vi "Load Reference.vi"(8 "error in (no error)":errorcluster, 10 "Reference":refnum<vi>, 11 "SingleStepTestV3 in":refnum<class "SingleStepTestV3.lvclass">) -> (0 "error out":errorcluster, 3 "SingleStepTestV3 out":refnum<class "SingleStepTestV3.lvclass">)   [LabVIEW 2022 SP3, in "SingleStepTestV3.lvlib" / "SingleStepTestV3.lvclass"]
doc: "The <b>Load Reference VI</b> is a dynamic dispatch VI that must be overwritten in every QControl Class and must <b>Call Parent Method</b>. This recursively loads the reference of the control to the data space for the Control Class up the inheritance hierarchy (class hierarchy). These references must be loaded in this way to use all of the built-in properties.\n\nThe reference input is the reference type needed for the control but is coerced to Generic. It should be cast back to the correct type before bundling into the class private data. The pre-casted \"Generic\" reference is wired as input to the <b>Call Parent Method</b>.\n<b> </b> <b> </b>\n©2016 Q Software Innovations, LLC (QSI)\nwritten by Quentin Alldredge\nproduced in LabVIEW 2015\n\nsupport@qsoftwareinnovations.com\nwww.qsoftwareinnovations.com\n\nAll rights reserved.\n\nRedistribution and use in source and binary forms, with or without modification, are permitted provided that the following conditions are met:\n\n * Redistributions of source code must retain the above copyright notice, this list of conditions and the following disclaimer.\n * Redistributions in binary form must reproduce the above copyright notice, this list of conditions and the following disclaimer in the documentation and/or other materials provided with the distribution.\n * Neither the name of Q Software Innovations, LLC. nor the names of its contributors may be used to endorse or promote products derived from this software without specific prior written permission.\n\nTHIS SOFTWARE IS PROVIDED BY THE COPYRIGHT HOLDERS AND CONTRIBUTORS \"AS IS\" AND ANY EXPRESS OR IMPLIED WARRANTIES, INCLUDING, BUT NOT LIMITED TO, THE IMPLIED WARRANTIES OF MERCHANTABILITY AND FITNESS FOR A PARTICULAR PURPOSE ARE DISCLAIMED. IN NO EVENT SHALL THE COPYRIGHT OWNER OR CONTRIBUTORS BE LIABLE FOR ANY DIRECT, INDIRECT, INCIDENTAL, SPECIAL, EXEMPLARY, OR CONSEQUENTIAL DAMAGES (INCLUDING, BUT NOT LIMITED TO, PROCUREMENT OF SUBSTITUTE GOODS OR SERVICES; LOSS OF USE, DATA, OR PROFITS; OR BUSINESS INTERRUPTION) HOWEVER CAUSED AND ON ANY THEORY OF LIABILITY, WHETHER IN CONTRACT, STRICT LIABILITY, OR TORT (INCLUDING NEGLIGENCE OR OTHERWISE) ARISING IN ANY WAY OUT OF THE USE OF THIS SOFTWARE, EVEN IF ADVISED OF THE POSSIBILITY OF SUCH DAMAGE."
uses:
  SingleStepTestV3.lvclass
  SingleStepTestV3.lvclass/SingleStepTestV3.ctl
  <vilib>/QSI/QControls/QControl Classes/Cluster/Cluster.lvclass
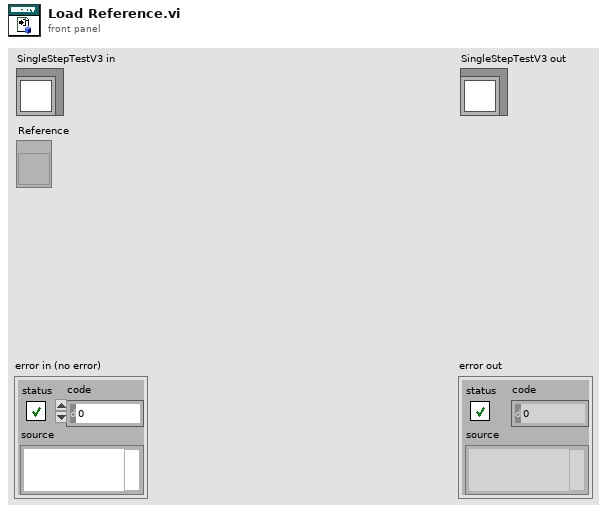
[diagram p1: front panel]
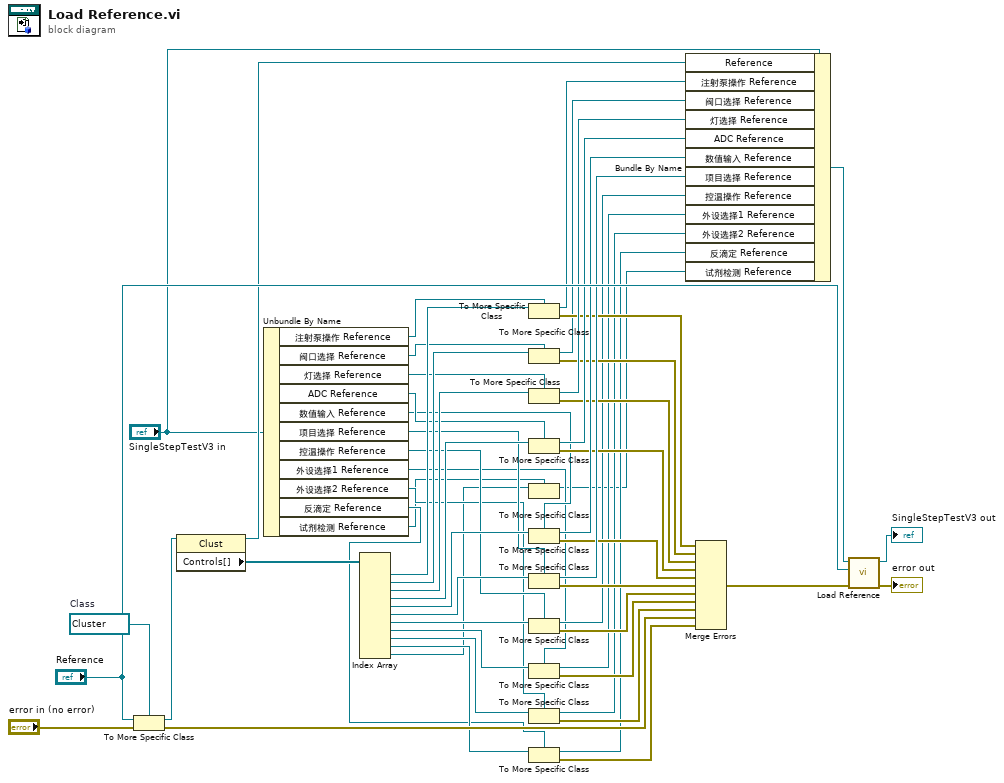
[diagram p0: block diagram]
diagram:
  w53 = refnum<vi> refnum  # Class
  n1 = To More Specific Class(target class=w53, reference="Reference", error in="error in (no error)") -> (specific class reference=w48:refnum<vi>, error out=w55:errorcluster)
  n2 = property class="Clust"(reference=w48) -> (reference out=w38:refnum<vi>, "Controls[]"=w47:refnum<vi>[])  [unwired: 1 in, 1 out]
  n3 = Unbundle By Name("SingleStepTestV3 in") -> ("注射泵操作 Reference"=w16:refnum<vi>, "阀口选择 Reference"=w15:refnum<vi>, "灯选择 Reference"=w14:refnum<vi>, "ADC Reference"=w13:refnum<vi>, "数值输入 Reference"=w12:refnum<vi>, "项目选择 Reference"=w11:refnum<vi>, "控温操作 Reference"=w10:refnum<vi>, "外设选择1 Reference"=w9:refnum<vi>, "外设选择2 Reference"=w8:refnum<vi>, "反滴定 Reference"=w6:refnum<vi>, "试剂检测 Reference"=w2:refnum<vi>)
  n4 = Index Array(array=w47) -> (element #1=w46:refnum<vi>, element #2=w45:refnum<vi>, element #3=w44:refnum<vi>, element #4=w42:refnum<vi>, element #5=w37:refnum<vi>, element #6=w36:refnum<vi>, element #7=w35:refnum<vi>, element #8=w34:refnum<vi>, element #9=w33:refnum<vi>, element #10=w7:refnum<vi>, element #11=w3:refnum<vi>)  [unwired: 11 in]
  n5 = To More Specific Class(target class=w16, reference=w46) -> (specific class reference=w22:refnum<vi>, error out=w23:errorcluster)  [unwired: 1 in]
  n6 = To More Specific Class(target class=w15, reference=w45) -> (specific class reference=w21:refnum<vi>, error out=w24:errorcluster)  [unwired: 1 in]
  n7 = To More Specific Class(target class=w14, reference=w44) -> (specific class reference=w43:refnum<vi>, error out=w25:errorcluster)  [unwired: 1 in]
  n8 = To More Specific Class(target class=w13, reference=w42) -> (specific class reference=w41:refnum<vi>, error out=w26:errorcluster)  [unwired: 1 in]
  n9 = To More Specific Class(target class=w2, reference=w3) -> (specific class reference=w1:refnum<vi>)  [unwired: 1 in, 1 out]
  n10 = To More Specific Class(target class=w12, reference=w37) -> (specific class reference=w40:refnum<vi>, error out=w27:errorcluster)  [unwired: 1 in]
  n11 = To More Specific Class(target class=w11, reference=w36) -> (specific class reference=w39:refnum<vi>, error out=w28:errorcluster)  [unwired: 1 in]
  n12 = To More Specific Class(target class=w10, reference=w35) -> (specific class reference=w20:refnum<vi>, error out=w29:errorcluster)  [unwired: 1 in]
  n13 = To More Specific Class(target class=w9, reference=w34) -> (specific class reference=w19:refnum<vi>, error out=w30:errorcluster)  [unwired: 1 in]
  n14 = To More Specific Class(target class=w8, reference=w33) -> (specific class reference=w18:refnum<vi>, error out=w31:errorcluster)  [unwired: 1 in]
  n15 = To More Specific Class(target class=w6, reference=w7) -> (specific class reference=w4:refnum<vi>, error out=w5:errorcluster)  [unwired: 1 in]
  n16 = Bundle By Name(cluster="SingleStepTestV3 in", "Reference"=w38, "注射泵操作 Reference"=w22, "阀口选择 Reference"=w21, "灯选择 Reference"=w43, "ADC Reference"=w41, "数值输入 Reference"=w40, "项目选择 Reference"=w39, "控温操作 Reference"=w20, "外设选择1 Reference"=w19, "外设选择2 Reference"=w18, "反滴定 Reference"=w4, "试剂检测 Reference"=w1) -> (w52:refnum<class "SingleStepTestV3.lvclass">)
  n17 = Merge Errors(w23, w24, w25, w26, w27, w28, w29, w30, w31, w55, w5) -> (w32:errorcluster)
  n18 = call-parent "Load Reference.vi"("error in (no error)"=w32, "Reference"="Reference", "Cluster in"=w52) -> ("error out"=→"error out":errorcluster, "Cluster out"=→"SingleStepTestV3 out":refnum<class "SingleStepTestV3.lvclass">)  [unwired: 7 in]
